vi "Drive Set Feet.vi"(1 "Feet":dbl=10.0 format="%#_13g", 2 "Direction":T1(ring)) -> (0 "Distance (ft)":dbl(knob) scale=0.0..10.0)   [LabVIEW 2014]
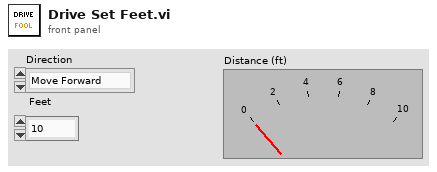
[diagram p1: front panel]
types:
  T1 = enum16{"Move Forward", "Move Backward", "Strafe Right", "Strafe Left"}
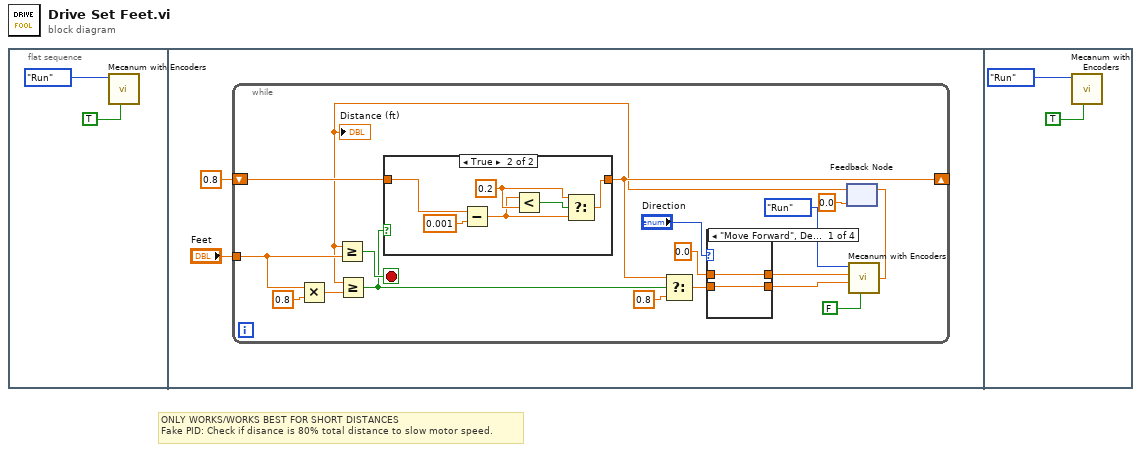
[diagram p0: block diagram]
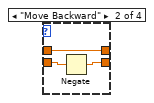
[diagram p3: hidden frame]
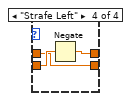
[diagram p5: hidden frame]
diagram:
  # "ONLY WORKS/WORKS BEST FOR SHORT DISTANCES\nFake PID: Check if disance is 80% total distance to slow motor speed."
  n1 = flat-sequence {
    frame #0 {
      n2 = call "Mecanum with Encoders.vi"("Reset"=TRUE, "Mode"=enum8{"Start", "Run", "Finish"}."Run") -> ()  [unwired: 4 in, 1 out]
    }
    frame #1 {
      n3 = while {
        tunnel: "Feet" -> [w18]
        shift-right: [w13] -> _
        shift-left: 0.8 -> [w14]
        stop <- w22 stop-if-true
        n4 = Multiply(x=w18, y=0.8) -> (x*y=w16:dbl)
        n5 = feedback #1(0.0 ("Distance (ft)")) -> (w6:dbl)
        "Distance (ft)" <- w6
        n6 = Greater Or Equal?(x=w6, y=w18) -> (x >= y?=w22:bool)
        n7 = Greater Or Equal?(x=w6, y=w16) -> (x >= y?=w12:bool)
        n8 = case shown="True" w12 {
          tunnel: w14 -> [w23 w28]
          tunnel: [w23 w24] -> w13
          frame False {
          }
          frame True {
            w26 = 0.2 ("y")
            n9 = Subtract(x=w28, y=0.001) -> (x-y=w25:dbl)
            n10 = Less?(x=w25, y=w26) -> (x < y?=w27:bool)
            n11 = Select(t=w26, s=w27, f=w25) -> (s? t:f=w24:dbl)
          }
        }
        n12 = Select(t=w13, s=w12, f=0.8) -> (s? t:f=w11:dbl)
        n13 = case shown="\"Move Forward\", Default" "Direction" {
          tunnel: w11 -> [w31 w34 w36 w39]
          tunnel: [w31 w33 w35 w37] -> w21
          tunnel: [w30 w32 w36 w38] -> w20
          tunnel: 0.0 ("Turn") -> [w30 w32 w35 w37]
          frame "Move Forward", Default {
          }
          frame "Move Backward" {
            n14 = Negate(x=w34) -> (-x=w33:dbl)
          }
          frame "Strafe Right" {
          }
          frame "Strafe Left" {
            n15 = Negate(x=w39) -> (-x=w38:dbl)
          }
        }
        n16 = call "Mecanum with Encoders.vi"("Reset"=FALSE, "Forward/Backward"=w21, "Strafe"=w20, "Mode"=enum8{"Start", "Run", "Finish"}."Run") -> ("Distance (ft)"=w7:dbl)  [unwired: 2 in]
        n17 = feedback-in #1(w7) -> ()
      }
    }
    frame #2 {
      n18 = call "Mecanum with Encoders.vi"("Reset"=TRUE, "Mode"=enum8{"Start", "Run", "Finish"}."Run") -> ()  [unwired: 4 in, 1 out]
    }
  }
